vi "OAT Output Buffered Data.vi"   [LabVIEW 2017, in "SoundVib_OAUtility.lvlib"]
doc: "Buffers the input signals and returns them in first-in first-out (FIFO) mode. Use <B>buffer settings</B> to set the buffer size and units. Each instance of this VI maintains its own state; use the N Waveforms instance of this VI to process an array of channels. Wire data to the <B>XY signal</B> input to determine the polymorphic instance to use or manually select the instance."
uses:
  <vilib>/addons/Sound and Vibration/Order Analysis/Utility/SoundVib_OAUtility.lvlib
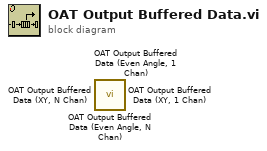
[diagram p0: block diagram]
diagram:
  n1 = call <vilib>:"OAT Output Buffered Data (Even Angle, N Chan).vi"() -> ()  [unwired: 13 in, 3 out]
  n2 = call <vilib>:"OAT Output Buffered Data (Even Angle, 1 Chan).vi"() -> ()  [unwired: 13 in, 3 out]
  n3 = call <vilib>:"OAT Output Buffered Data (XY, N Chan).vi"() -> ()  [unwired: 13 in, 3 out]
  n4 = call <vilib>:"OAT Output Buffered Data (XY, 1 Chan).vi"() -> ()  [unwired: 13 in, 3 out]
